vi "Display_IP_Addresses.vi"(8 "Error In":errorcluster, 11 "Data":T1={"Info Box"="", "MAC & Name Out"=[], "Default Gateway"="", "Drfiter IP Addresses"=[], "Network Map"="", "Drifter Selection"=0, "File Selection"=0, "Download File Path"=path "", "File Selection Strings"=[], "Sample Rate"=enum." 0.2", "Log While Charging"=enum." Yes"}) -> (0 "Error Out":errorcluster, 2 "Menu String":string[](array[string]), 3 "Output Text":string)   [LabVIEW 2017]
uses:
  data.ctl
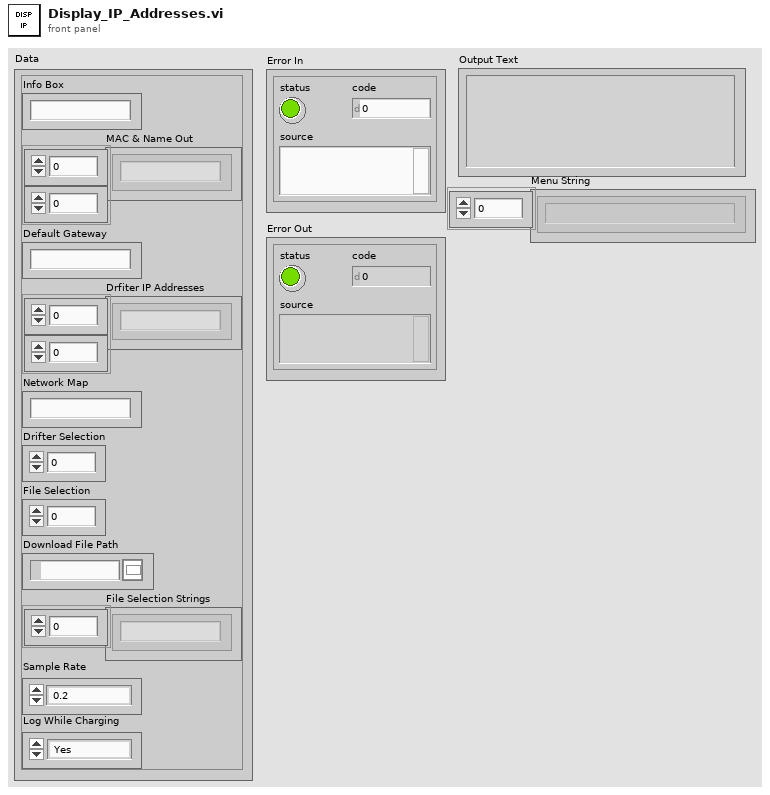
[diagram p1: front panel]
types:
  T1 = typedef "data.ctl" = cluster{"Info Box":string, "MAC & Name Out":string[][], "Default Gateway":string, "Drfiter IP Addresses":string[][], "Network Map":string, "Drifter Selection":i32, "File Selection":i32, "Download File Path":path, "File Selection Strings":string[], "Sample Rate":enum32{"No Selection", " 0.2", " 0.1", " 1", " 2", " 5", " 10"}, "Log While Charging":enum32{"No Selection", " Yes", " No"}}
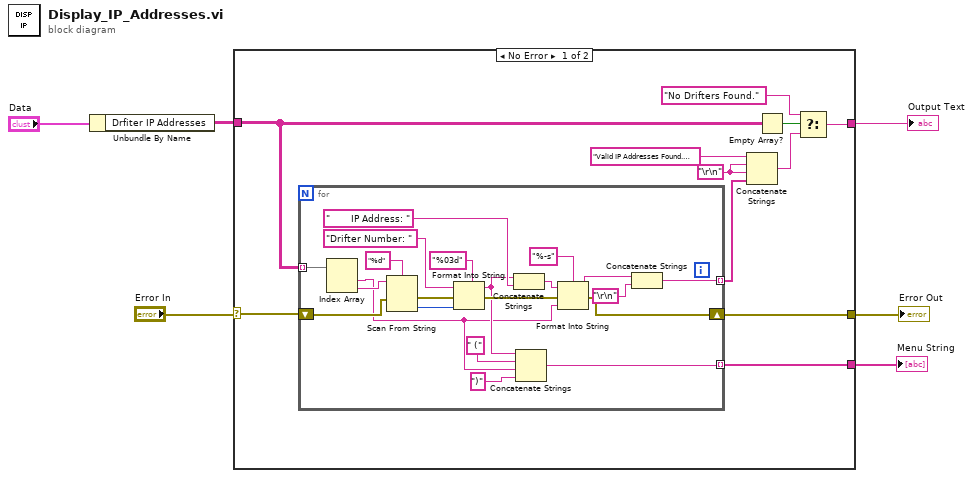
[diagram p0: block diagram]
diagram:
  n1 = Unbundle By Name("Data") -> ("Drfiter IP Addresses"=w6:string[][])
  n2 = case shown="No Error" "Error In" {
    selector: "Error In" -> [w10 w39]
    tunnel: w6 -> [w11 _]
    tunnel: [w9 w39] -> w4
    tunnel: [w8 _] -> w3
    tunnel: [w7 _] -> w2
    frame No Error {
      w13 = "\r\n"
      n3 = for {
        tunnel: w11 -> [w38] mode=indexing
        tunnel: [w37] -> w12 mode=indexing
        shift-right: [w23] -> w9
        shift-left: w10 -> [w32]
        tunnel: [w18] -> w7 mode=indexing
        n4 = Index Array(array=w38) -> (element #1=w20:string, element #2=w25:string)  [unwired: 2 in]
        n5 = Scan From String(format string="%d", input string=w25, error in=w32) -> (error out=w31:errorcluster, output 1=w33:i32)  [unwired: 2 in, 2 out]
        n6 = Format Into String(format string="%03d", initial string="Drifter Number: " ("string"), error in=w31, w33) -> (resulting string=w22:string, error out=w30:errorcluster)
        n7 = Concatenate Strings(w22, "       IP Address: " ("string")) -> (w28:string)
        n8 = Concatenate Strings(w22, " (" ("string"), w20, ")" ("string")) -> (w18:string)
        n9 = Format Into String(format string="%-s", initial string=w28, error in=w30, w20) -> (resulting string=w26:string, error out=w23:errorcluster)
        n10 = Concatenate Strings(w26, "\r\n") -> (w37:string)
      }
      n11 = Concatenate Strings("Valid IP Addresses Found. Select a drifter from the drop-down menu and press \"List Data Files\" to display its data files:", w13, w13, w12) -> (w15:string)
      n12 = Empty Array?(array=w11) -> (empty?=w17:bool)
      n13 = Select(t="No Drifters Found.", s=w17, f=w15) -> (s? t:f=w8:string)
    }
    frame Error {
    }
  }
  "Output Text" <- w3
  "Error Out" <- w4
  "Menu String" <- w2
